vi "Robot Global Data.vi"() -> ()   [LabVIEW 2015]
doc: "This global VI can contain as many global variables as you need. Place a control on the panel, give it a good name. To read or write to it from a VI, drag the icon to the diagram of that VI. You can also drag from the project. Click on the node to change which global you access. You shouldn't have multiple locations writing to a global or it will cause a race-condition."
uses:
  <vilib>/Rock Robotics/WPI/DriverStation/WPI_DriverStationRobotMode2.ctl
  <vilib>/Rock Robotics/WPI/Camera/WPI_CameraImageSize.ctl
panel:
  in  "Tab Control":T1(tab)=enum."Preferences"
  in  "Enable IR Seeker":bool=TRUE
  in  "Enable LED 2":bool=TRUE
  in  "Enable LED 1":bool=TRUE
  in  "Enable Optical Distance":bool=TRUE
  in  "Enable Push Button 2":bool=TRUE
  in  "Enable Push Button 1":bool=TRUE
  in  "Enable Potentiometer R":bool=TRUE
  in  "Enable Potentiometer L":bool=TRUE
  in  "Enable Servo 2":bool=TRUE
  in  "Enable Servo 1":bool=TRUE
  in  "Enable Compressor":bool=TRUE
  in  "Enable Target Vision":bool
  in  "Enable Catapult":bool
  in  "Enable Ball Holder":bool
  in  "Enable Ball Loader Rollers":bool
  in  "Enable Ball Loader Lift":bool
  in  "Enable Drive Wheels":bool=TRUE
  in  "Enable Xbox 1":bool=TRUE
  in  "Enable Xbox 0":bool=TRUE
  in  "Enable PCM":bool
  in  "Enable PDP":bool
  in  "Enable Gyro":bool=TRUE
  in  "Enable TTL Display":bool=TRUE
  in  "Enable RGB Sensor":bool=TRUE
  in  "Enable I2C TC74":bool=TRUE
  in  "Enable MCP9808":bool=TRUE
  in  "Enable Wheel Encoders":bool
  in  "Enable I2C Accelerometer":bool=TRUE
  in  "Enable I2C Display":bool=TRUE
  in  "Enable Accelerometer":bool=TRUE
  in  "Enable Drive Vision":bool
  in  "I2C Display 2":u16=2016
  in  "Drive Kf Gain":dbl=0.5 format="%.4g"
  in  "Autonomous Mode":i8
  in  "Drive Kd Gain":dbl format="%.4g"
  in  "Drive Ki Gain":dbl=0.0001 format="%.4g"
  in  "Drive Kp Gain":dbl=0.0005 format="%.4g"
  in  "Lift Kf Gain":dbl format="%.4g"
  in  "Lift Kd Gain":dbl format="%.4g"
  in  "Lift Ki Gain":dbl=0.02 format="%.4g"
  in  "Lift Kp Gain":dbl=1.0 format="%.4g"
  in  "I2C Display 1":u16=3960
  in  "Brightness":u8(knob)=5 scale=0.0..15.0
  in  "Blink Display":bool
  in  "Robot Mode":T2=enum."Finish"
  in  "Pick-Up Roller Gain":dbl(slide)=0.5050505050505051 scale=0.0..1.0
  in  "Ball Holder Gain":dbl(slide)=0.5050505050505051 scale=0.0..1.0
  out "X-Acceleration Ext":dbl format="%#_2g"
  out "Y-Acceleration Ext":dbl format="%#_2g"
  out "Z-Acceleration Ext":dbl format="%#_2g"
  out "RGB Blue":u16
  out "RGB Green":u16
  out "RGB Red":u16
  out "RGB Clear":u16
  out "Right Pot":dbl format="%.2f"
  out "Left Pot":dbl format="%.2f"
  in  "Yaw (Radians)":dbl=0.008209159386752757 format="%#_4g"
  out "Optical Distance":dbl=2.6342770740000003 format="%.2g"
  out "Gyro Cal":dbl=2.454 format="%.3f"
  in  "Accelerometer Gain":dbl=1.0 format="%.4g"
  in  "Gyro Gain":dbl=0.0125 format="%.4f"
  out "Gyro Temp":dbl format="%.2f"
  out "Gyro Angle":dbl=0.47035018621113606 format="%.2f"
  out "Gyro Rate":dbl=0.013828276171874999 format="%.2f"
  out "Comp Current":dbl format="%.2f"
  out "PCM Voltage":dbl format="%.2f"
  out "Battery Current":dbl format="%.2f"
  out "Right Track Rate":dbl format="%.2g"
  out "Left Track Rate":dbl format="%.2g"
  out "Right Track Position":dbl format="%.2g"
  out "Left Track Position":dbl format="%.2g"
  out "Battery Voltage":dbl format="%.2f"
  out "Z-Acceleration":dbl=1.001953125 format="%.3f"
  out "Y-Acceleration":dbl=0.01171875 format="%.3f"
  out "X-Acceleration":dbl=-0.009765625 format="%.3f"
  out "Seeker Direction":u8
  out "Seeker ID":u8
  out "Seeker Manufacturer":u8
  out "Seeker Firmware":u8
  out "Temperature 2":dbl(slide) scale=0.0..100.0
  out "Temperature 1":u8(slide) scale=0.0..100.0
  in  "LED 2":bool
  in  "LED 1":bool
  in  "Servo 2 Position":i32(slide)=85 scale=0.0..170.0
  in  "Servo 1 Position":i32(slide)=85 scale=0.0..170.0
  in  "Pot R Position":dbl(knob)=0.5012424699086809 scale=0.0..1.0
  out "Push Button 4":bool
  out "Push Button 3":bool
  out "Push Button 2":bool
  in  "Pot L Position":dbl(knob)=0.4988640617378445 scale=0.0..1.0
  out "Push Button 1":bool
  out "Xbox 1 - POV":dbl
  in  "Xbox 1 - Right Trigger":dbl(slide) scale=-1.0..1.0
  in  "Xbox 1 - Left Trigger":dbl(slide) scale=-1.0..1.0
  in  "Xbox 1 - Right Thumb X":dbl(slide) scale=-1.0..1.0
  in  "Xbox 1 - Right Thumb Y":dbl(slide) scale=1.0..-1.0
  out "Xbox 1 - Button Right Thumb":bool
  out "Xbox 1 - Button Left Thumb":bool
  out "Xbox 1 - Button Start":bool
  out "Xbox 1 - Button Back":bool
  out "Xbox 1 - Button RB":bool
  out "Xbox 1 - Button LB":bool
  out "Xbox 1 - Button Y":bool
  out "Xbox 1 - Button X":bool
  out "Xbox 1 - Button B":bool
  out "Xbox 1 - Button A":bool
  in  "Xbox 1 - Left Thumb X":dbl(slide) scale=-1.0..1.0
  in  "Xbox 1 - Left Thumb Y":dbl(slide) scale=1.0..-1.0
  out "Xbox 0 - POV":dbl
  in  "Xbox 0 - Right Trigger":dbl(slide) scale=-1.0..1.0
  in  "Xbox 0 - Left Trigger":dbl(slide) scale=-1.0..1.0
  in  "Xbox 0 - Right Thumb X":dbl(slide)=0.047244094488188976 scale=-1.0..1.0
  in  "Xbox 0 - Right Thumb Y":dbl(slide) scale=1.0..-1.0
  out "Xbox 0 - Button Right Thumb":bool
  out "Xbox 0 - Button Left Thumb":bool
  out "Xbox 0 - Button Start":bool
  out "Xbox 0 - Button Back":bool
  out "Xbox 0 - Button RB":bool
  out "Xbox 0 - Button LB":bool
  out "Xbox 0 - Button Y":bool
  out "Xbox 0 - Button X":bool
  out "Xbox 0 - Button B":bool
  out "Xbox 0 - Button A":bool
  in  "Xbox 0 - Left Thumb X":dbl(slide)=0.05511811023622047 scale=-1.0..1.0
  in  "Xbox 0 - Left Thumb Y":dbl(slide)=-0.07086614173228346 scale=1.0..-1.0
  out "Local RT X":dbl
  out "Local LT Y":dbl
  out "Case":u16
  out "Translation":bool
  out "Rotation":bool
  out "Right Encoder Count":dbl=285122.0
  out "Left Encoder Count":dbl=-7784132.0
  in  "Drivetrain Mode":u16
  out "FR Overcurrent Counter":u8(slide) scale=0.0..5.0
  out "FR Lift Overcurrent Error":bool
  out "Right Drive Current":dbl(knob)=0.125 scale=0.0..30.0
  out "FR Lift Lower Limit":bool
  out "FR Lift Upper Limit":bool
  in  "FR Lift Encoder Position":dbl(slide) scale=0.0..48.0
  out "FL Lift Overcurrent Error":bool
  out "Left Drive Current":dbl(knob)=0.25 scale=0.0..30.0
  in  "FL Lift Encoder Position":dbl(slide) scale=0.0..48.0
  out "FL Lift Lower Limit":bool
  out "FL Lift Upper Limit":bool
  out "FL Overcurrent Counter":u8(slide) scale=0.0..5.0
  in  "Front Lift Rate":dbl=150.0 format="%.2f"
  in  "Front Encoder Gain":dbl=400.0 format="%.2f"
  in  "Front Lift Limit":dbl=19000.0 format="%.2f"
  in  "Drive Vision Image Size":T3=enum."160x120"
  in  "Target Vision Image Size":T3=enum."160x120"
  out "Frames Per Second":dbl=20.0
  in  "Minimum Score Treshold":dbl=75.0
  out "Target Acquired":bool
  in  "Active Dashboard Camera":dbl
  out "Processing Time (ms)":u32=50
  out "Detected Targets":T4(array[cluster]) {"Normalized Rect"."Numeric 5" format="%#_2g"; "Normalized Rect"."Numeric 3" format="%#_2g"; "Normalized Rect"."Numeric 2" format="%#_2g"; "Normalized Rect"."Numeric" format="%#_2g"}
  # "I/O Definitions"
  # "PWM OUTPUTS\nPWM 0 - \nPWM 1 - \nPWM 2 - \nPWM 3 - \nPWM 4 - \nPWM 5 - \nPWM 6 - \nPWM 7 - \nPWM 8 - \nPWM 9 - \n\nRELAY OUTPUTS\nRELAY 0 = \nRELAY 1 = \nRELAY 2 = \nRELAY 3 = \n\nSOLENOID OUTPUTS\nDO 1 = \nDO 2 = \nDO 3 = \nDO 4 = \nDO 5 = \nDO 6 = \nDO 7 = \nDO 8 =\n\nANALOG INPUTS\nAI 0 = Yaw Gyro\nAI 1 = \nAI 2 = \nAI 3 = \n\nANALOG OUTPUTS\nAO 1 = \nAO2 ="
  # "DIGITAL I/O\nDIO 0 = \nDIO 1 = \nDIO 2 = \nDIO 3 = \nDIO 4 = \nDIO 5 = \nDIO 6 = \nDIO 7 = \nDIO 8 = \nDIO 9 = \n\nCAN BUS\nCAN   0 = Left Drivetrain Slave Motor Controller \nCAN   1 = Left Drivetrain Master Motor Controller\nCAN   2 = Right Drivetrain Master Motor Controller\nCAN   3 = Right Drivetrain Slave Motor Controller\nCAN   4 = Power Distribution Panel (PDP) \nCAN   5 = Linear Actuator\nCAN   6 = Pneumatics Control Module (PCM)\nCAN   7 = \nCAN   8 = \nCAN   9 =\nCAN 10 = \nCAN 11 = \nCAN 12 = \nCAN 13 = \nCAN 14 = \nCAN 15 = \n\nI2C ADDRESSES\n0x32 -> 0x33 = Accelerometer X Axis\n0x34 -> 0x35 = Accelerometer Y Axis\n0x36 -> 0x37 = Accelerometer Z Axis\n\nETHERNET ADDRESSES\n10.39.60.1 ="
  # "Sub-System Enablers"
  # "Preferences"
  # "Lift Gains"
  # "Drive Gains"
  # "Sensor Data"
  # "Sensor Data"
  # "Human - Machine Interface"
  # "Xbox 1\nController"
  # "Xbox 0\nController"
  # "Right Drive"
  # "LIMIT"
  # "LIMIT"
  # "CURRENT"
  # "Left Drive"
  # "LIMIT"
  # "LIMIT"
  # "CURRENT"
  # "Vision & Target Acquisition"
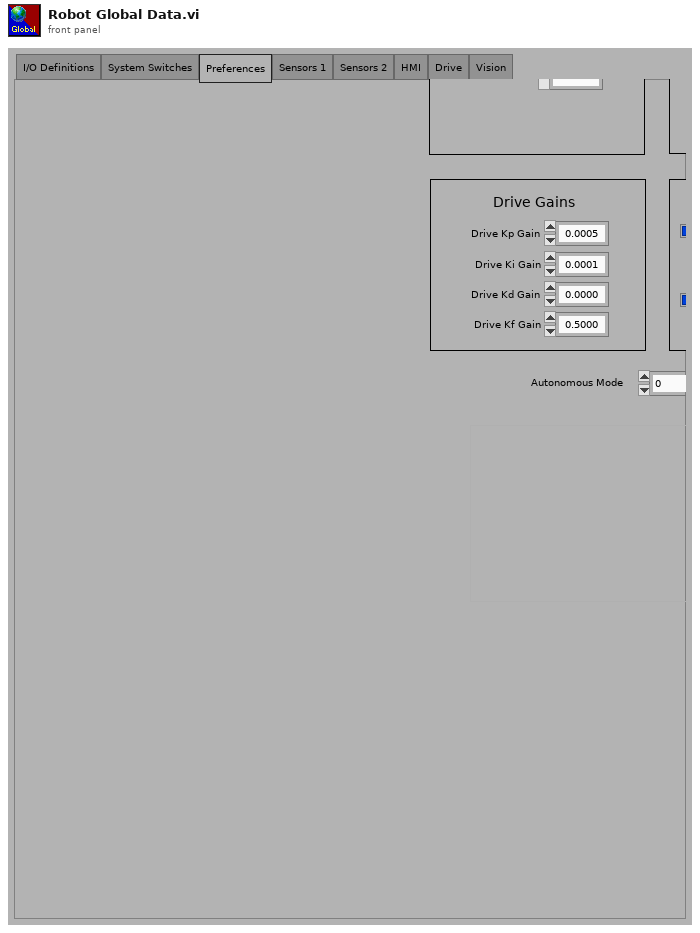
[diagram p1: front panel]
types:
  T1 = enum32{"I/O Definitions", "System Switches", "Preferences", "Sensors 1", "Sensors 2", "HMI", "Drive", "Vision"}
  T2 = typedef "WPI_DriverStationRobotMode2.ctl" = enum16{"Autonomous Disabled", "Autonomous Enabled", "Teleop Disabled", "Teleop Enabled", "Disconnected", "Finish", "Test Disabled", "Test Enabled", "Emergency Stopped"}
  T3 = typedef "WPI_CameraImageSize.ctl" = enum16{"640x480", "320x240", "160x120", "Custom"}
  T4 = cluster{"Distance (ft)":dbl, "Center":cluster{dbl, dbl}, "Normalized Rect":cluster{"Numeric":dbl, "Numeric 2":dbl, "Numeric 3":dbl, "Numeric 5":dbl}}[]
diagram:
